vi "Actor Template-Core_Initialize.vi"(0 "Initialization Sequence":string, 5 "FTW Actor Instance Configuration":string, 11 "error in (no error)":errorcluster) -> (4 "Actor Template-Core out":refnum<class "Actor Template-Core.lvclass">, 6 "Incoming Requests":refnum<event-registration>, 15 "error out":errorcluster)   [LabVIEW 2013, in "Actor Template-Core.lvclass"]
uses:
  Actor Template-Core.lvclass
  src/Message/Request/FTW-Message-IncomingRequest.lvclass
  Actor Template-Core.lvclass/Actor Template-Core.ctl
  Core/src/Reflection/FTW-Reflection-Type.vi
  Core/src/JSON/FTW-JSON-Core-LibraryFilepath.vi
  Core/src/JSON/FTW-JSON-Core-GetFlattenedValue.vi
  Core/src/JSON/FTW-JSON-Core-LibraryError.vi
  Core/utils/CodeGen/JSON Deserialize/FTW-JSON-Deserialize.xnode
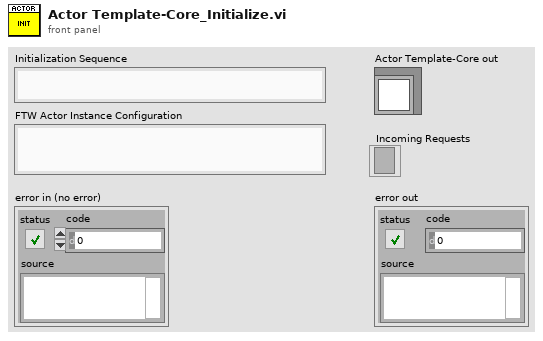
[diagram p1: front panel]
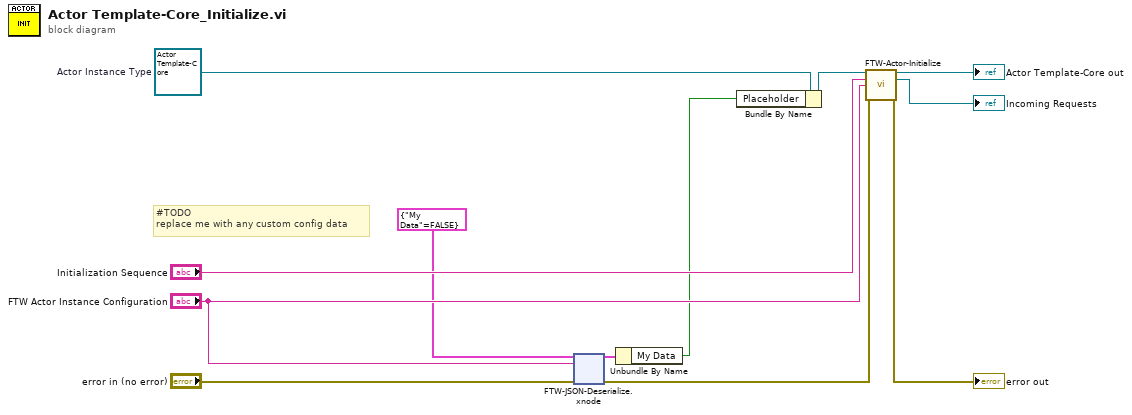
[diagram p0: block diagram]
diagram:
  w10 = refnum<class "Actor Template-Core.lvclass"> refnum  # Actor Instance Type
  # "#TODO\nreplace me with any custom config data"
  n1 = xnode "FTW-JSON-Deserialize.xnode"("Type and Defaults"=cluster{"My Data":bool} {"My Data"=FALSE}, "JSON String"="FTW Actor Instance Configuration", "error in"="error in (no error)") -> ("Values"=w2:cluster{"My Data":bool}, "error out"=w6:errorcluster)
  n2 = Unbundle By Name(w2) -> ("My Data"=w1:bool)
  n3 = Bundle By Name(cluster=w10, "Placeholder"=w1) -> (w3:refnum<class "Actor Template-Core.lvclass">)
  n4 = call-dynamic "FTW-Actor-Initialize.vi"("FTW Actor Instance Type"=w3, "Initialization Job Sequence"="Initialization Sequence", "Actor Instance Configuration"="FTW Actor Instance Configuration", "error in"=w6) -> ("FTW Actor Instance"=→"Actor Template-Core out":refnum<class "Actor Template-Core.lvclass">, "Incoming Requests"=→"Incoming Requests":refnum<event-registration>, "error out"=→"error out":errorcluster)  [unwired: 9 in]
